vi "Teleop_Get_DrivingMode.vi"() -> (3 "DrivingMode":i32)   [LabVIEW 2019]
uses:
  Teleop_Globals.vi
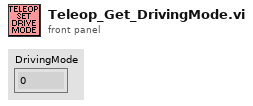
[diagram p1: front panel]
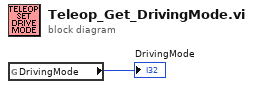
[diagram p0: block diagram]
diagram:
  n1 = global read "Teleop_Globals.vi" "DrivingMode"() -> (→"DrivingMode":i32)
